vi "QCP_WriteFile.vi"(6 "Overrite?":bool, 8 "error in":errorcluster, 9 "Path relative?":bool, 10 "Path":string, 11 "QCP_DevRef_In":T1) -> (0 "error out":errorcluster, 3 "QCP_DevRef_Out":T1)   [LabVIEW 2016]
uses:
  <userlib>/836-libraries/System/QCPv2/QCPSupportCode/QCP_RefNum.ctl
  <userlib>/836-libraries/System/QCPv2/QCPSupportCode/QCPData.ctl
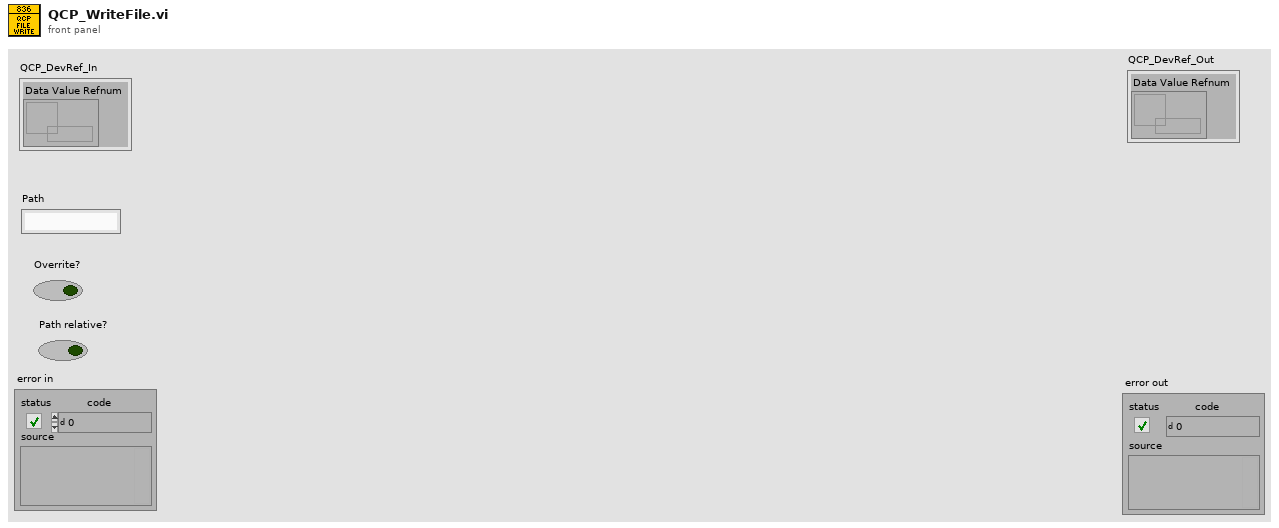
[diagram p1: front panel]
types:
  T1 = typedef "QCP_RefNum.ctl" = cluster{"Data Value Refnum":refnum<data-value>}
  T2 = enum16{"open", "replace", "create", "open or create", "replace or create", "replace or create with confirmation"}
  T3 = typedef "QCPData.ctl" = cluster{"Names":string[], "Values":cluster{"Array":dbl[]}[]}
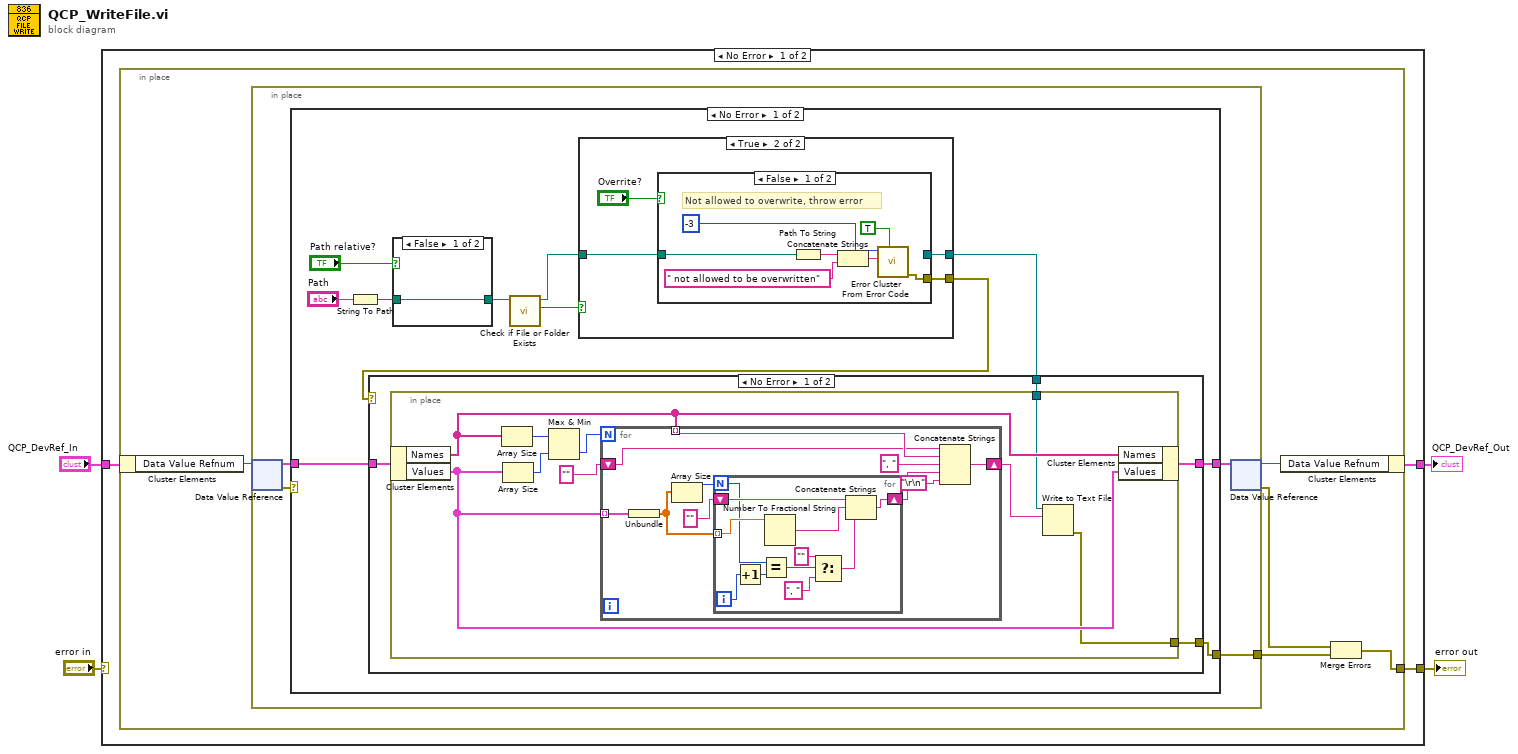
[diagram p0: block diagram]
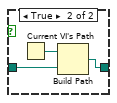
[diagram p3: hidden frame]
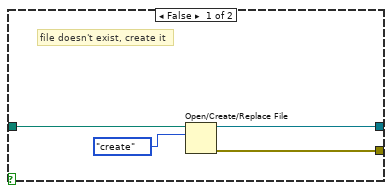
[diagram p4: hidden frame]
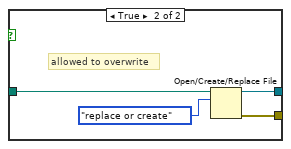
[diagram p5: hidden frame]
diagram:
  n1 = case shown="No Error" "error in" {
    selector: "error in" -> [_ w90]
    tunnel: [w6 w90] -> w3
    tunnel: "QCP_DevRef_In" -> [w7 w89]
    tunnel: [w5 w89] -> w1
    frame No Error {
      n2 = in-place {
        in-place-border: [w9] -> w6
        n3 = in-place-cluster #1(w7) -> ("Data Value Refnum"=w12:refnum<data-value>)
        n4 = in-place {
          in-place-border: [w14] -> w10
          n5 = in-place-dvr #2(w12) -> (w15:T3, w16:errorcluster)
          n6 = case shown="No Error" w16 {
            selector: w16 -> [_ w88]
            tunnel: w15 -> [w20 w87]
            tunnel: [w19 w88] -> w14
            tunnel: [w18 w87] -> w13
            frame No Error {
              n7 = String To Path(string="Path") -> (path=w26:path)
              n8 = case shown="False" "Path relative?" {
                tunnel: w26 -> [w64 w67]
                tunnel: [w64 w65] -> w27
                frame False {
                }
                frame True {
                  n9 = Current VI's Path() -> (path=w66:path)
                  n10 = Build Path(base path=w66, name or relative path=w67) -> (appended path=w65:path)
                }
              }
              n11 = call <vilib>:"Check if File or Folder Exists.vi"("path"=w27) -> ("file or folder exists?"=w22:bool, "dup path"=w23:path)  [unwired: 8 in, 1 out]
              n12 = case shown="True" w22 {
                tunnel: w23 -> [w71 w74]
                tunnel: [w69 w73] -> w21
                tunnel: [w70 w72] -> w17
                frame False {
                  # "file doesn't exist, create it"
                  n13 = Open/Create/Replace File(file path (use dialog)=w71, operation (0:open)=T2."create") -> (refnum out=w70:refnum<file>, error out=w69:errorcluster)  [unwired: 4 in, 1 out]
                }
                frame True {
                  n14 = case shown="False" "Overrite?" {
                    tunnel: w74 -> [w82 w85]
                    tunnel: [w80 w83] -> w73
                    tunnel: [_ w84] -> w72
                    frame False {
                      # "Not allowed to overwrite, throw error"
                      n15 = Path To String(path=w82) -> (string=w81:string)
                      n16 = Concatenate Strings(w81, " not allowed to be overwritten") -> (w77:string)
                      n17 = call <vilib>:"Error Cluster From Error Code.vi"("show call chain? (False)"=TRUE, "error message (\"\")"=w77, "error code (0)"=-3) -> ("error out"=w80:errorcluster)  [unwired: 6 in]
                    }
                    frame True {
                      # "allowed to overwrite"
                      n18 = Open/Create/Replace File(file path (use dialog)=w85, operation (0:open)=T2."replace or create") -> (refnum out=w84:refnum<file>, error out=w83:errorcluster)  [unwired: 4 in, 1 out]
                    }
                  }
                }
              }
              n19 = case shown="No Error" w21 {
                selector: w21 -> [_ w63]
                tunnel: w20 -> [w31 w62]
                tunnel: [w29 w63] -> w19
                tunnel: [w30 w62] -> w18
                tunnel: w17 -> [w28 _]
                frame No Error {
                  n20 = in-place {
                    in-place-border: [w34] -> w29
                    in-place-border: w28 -> [w33]
                    n21 = in-place-cluster #3(w31) -> ("Names"=w36:string[], "Values"=w35:cluster{"Array":dbl[]}[])
                    n22 = Array Size(array=w36) -> (size(s)=w39:i32)
                    n23 = Array Size(array=w35) -> (size(s)=w40:i32)
                    n24 = Max & Min(x=w39, y=w40) -> (min(x,y)=w38:i32)  [unwired: 1 out]
                    n25 = for {
                      N: w38 -> [_]
                      tunnel: w36 -> [w50] mode=indexing
                      tunnel: w35 -> [w48] mode=indexing
                      shift-right: [w44] -> w32
                      shift-left: "" -> [w42]
                      n26 = Unbundle(w48) -> ("Array"=w46:dbl[])
                      n27 = Array Size(array=w46) -> (size(s)=w47:i32)
                      n28 = for {
                        N: w47 -> [w53]
                        tunnel: w46 -> [w61] mode=indexing
                        shift-right: [w60] -> w41
                        shift-left: "" -> [w59]
                        i -> [w55]
                        n29 = Increment(x=w55) -> (x+1=w54:i32)
                        n30 = Equal?(x=w53, y=w54) -> (x = y?=w57:bool)
                        n31 = Number To Fractional String(number=w61) -> (F-format string=w58:string)  [unwired: 3 in]
                        n32 = Select(t="", s=w57, f=", ") -> (s? t:f=w56:string)
                        n33 = Concatenate Strings(w59, w58, w56) -> (w60:string)
                      }
                      n34 = Concatenate Strings(w42, w50, ", " ("string"), w41, "\r\n") -> (w44:string)
                    }
                    n35 = Write to Text File(file (use dialog)=w33, text=w32) -> (error out=w34:errorcluster)  [unwired: 2 in, 2 out]
                    n36 = in-place-cluster #3("Names"=w36, "Values"=w35) -> (w30:T3)
                  }
                }
                frame Error {
                }
              }
            }
            frame Error {
            }
          }
          n37 = in-place-dvr #2(w13) -> (w11:refnum<data-value>, w8:errorcluster)
        }
        n38 = in-place-cluster #1("Data Value Refnum"=w11) -> (w5:T1)
        n39 = Merge Errors(w8, w10) -> (w9:errorcluster)
      }
    }
    frame Error {
    }
  }
  "QCP_DevRef_Out" <- w1
  "error out" <- w3
